vi "Save Data _ Create File.vi"(8 "error in":errorcluster) -> (0 "error out":errorcluster, 1 "FiileNote":string, 2 "FileName":string, 3 "file out":refnum<k34>)   [LabVIEW 2016]
uses:
  Ctrls/GlobeVaribles.vi
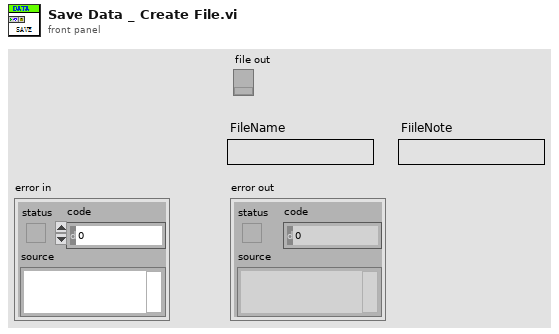
[diagram p1: front panel]
types:
  T1 = enum16{"open", "open or create", "create or replace", "create", "open (read-only)"}
  T2 = typedef "Global para Config.ctl" = cluster{"Timing":cluster{"SampleRate":i32}, "SavePara":cluster{"FlowDiskMode":T3, "SelectMode":T4, "FolderPath":path, "Filename":string, "FileNote":string, "AutoInterval":i32, "Template":path}, "ConfigDS Path*":path, "Tdms Ref*":refnum<k34>}
  T3 = typedef "File Save Mode.ctl" = i32
  T4 = typedef "Select Point Mode.ctl" = i32
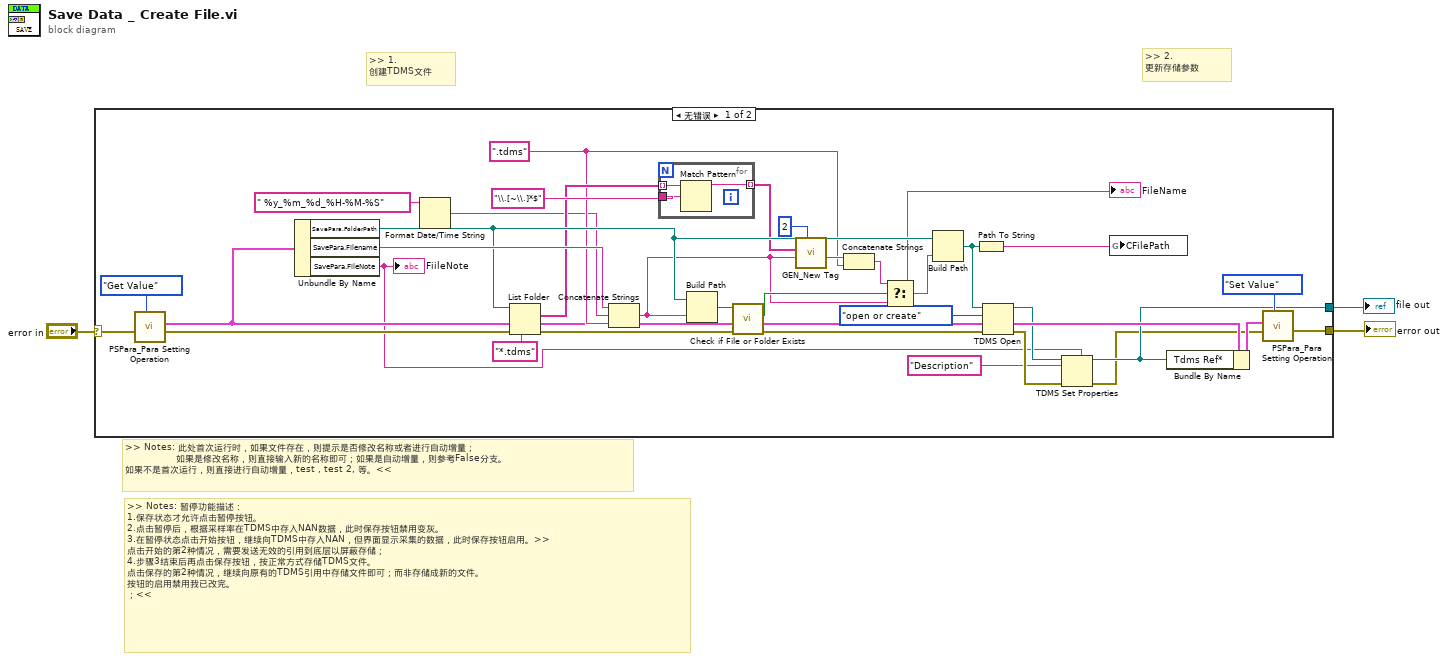
[diagram p0: block diagram]
diagram:
  # ">> 2.\n更新存储参数"
  # ">> 1.\n创建TDMS文件"
  # ">> Notes: 暂停功能描述：\n1.保存状态才允许点击暂停按钮。\n2.点击暂停后，根据采样率在TDMS中存入NAN数据，此时保存按钮禁用变灰。\n3.在暂停状态点击开始按钮，继续向TDMS中存入NAN，但界面显示采集的数据，此时保存按钮启用。>>\n点击开始的第2种情况，需要发送无效的引用到底层以屏蔽存储；\n4.步骤3结束后再点击保存按钮，按正常方式存储TDMS文件。\n点击保存的第2种情况，继续向原有的TDMS引用中存储文件即可；而非存储成新的文件。\n按钮的启用禁用我已改完。\n；<<"
  # ">> Notes: 此处首次运行时，如果文件存在，则提示是否修改名称或者进行自动增量；\n                 如果是修改名称，则直接输入新的名称即可；如果是自动增量，则参考False分支。\n如果不是首次运行，则直接进行自动增量，test , test 2, 等。<<"
  n1 = case shown="无错误" "error in" {
    selector: "error in" -> [w34 w41]
    tunnel: [w37 w41] -> w1
    tunnel: [w8 _] -> w2
    frame No Error {
      w14 = ".tdms" ("字符串")
      n2 = call "PSPara_Para Setting Operation.vi"("Operation"=enum16{"Set Value", "Get Value", "Initialize"}."Get Value", "error in"=w34) -> ("error out"=w33:errorcluster, "_Para"=w10:T2)  [unwired: 8 in]
      n3 = Unbundle By Name(w10) -> ("SavePara.FolderPath"=w35:path, "SavePara.Filename"=w36:string, "SavePara.FileNote"=w5:string)
      "FiileNote" <- w5
      n4 = Format Date/Time String(time format string (%c)=" %y_%m_%d_%H-%M-%S") -> (date/time string=w13:string)  [unwired: 2 in]
      n5 = List Folder(path=w35, pattern="*.tdms", error in=w33) -> (filenames=w24:string[], error out=w16:errorcluster)  [unwired: 1 in, 2 out]
      n6 = Concatenate Strings(w36, w13, w14) -> (w11:string)
      n7 = for {
        tunnel: "\\.[~\\.]*$" ("regular expression") -> [w40]
        tunnel: w24 -> [w39] mode=indexing
        tunnel: [w38] -> w23 mode=indexing
        n8 = Match Pattern(string=w39, regular expression=w40) -> (before substring=w38:string)  [unwired: 4 out]
      }
      n9 = Build Path(base path=w35, name or relative path=w11) -> (appended path=w22:path)
      n10 = call <vilib>:"Check if File or Folder Exists.vi"("error in (no error)"=w16, "path"=w22) -> ("error out"=w15:errorcluster, "file or folder exists?"=w21:bool)  [unwired: 7 in, 1 out]
      n11 = call "GEN_New Tag.vi"("Start Point"=2, "Basic"=w11, "Exist"=w23) -> ("Name"=w29:string)  [unwired: 7 in, 1 out]
      n12 = Concatenate Strings(w29, w14) -> (w20:string)
      n13 = Select(t=w20, s=w21, f=w11) -> (s? t:f=w19:string)
      "FileName" <- w19
      n14 = Build Path(base path=w35, name or relative path=w19) -> (appended path=w18:path)
      n15 = Path To String(path=w18) -> (string=w17:string)
      n16 = TDMS Open(8:w15, 10:T1."open or create" ("operation (0:open)"), 11:w18) -> (0:w7:errorcluster, 3:w9:refnum<k34>)  [unwired: 4 in]
      n17 = TDMS Set Properties(5:w5, 7:"Description", 8:w7, 11:w9) -> (0:w6:errorcluster, 3:w8:refnum<k34>)  [unwired: 2 in, 2 out]
      n18 = global write "GlobeVaribles.vi" "CFilePath"(w17) -> ()
      n19 = Bundle By Name(cluster=w10, "Tdms Ref*"=w8) -> (w31:T2)
      n20 = call "PSPara_Para Setting Operation.vi"("Operation"=enum16{"Set Value", "Get Value", "Initialize"}."Set Value", "error in"=w6, "_Para"=w31) -> ("error out"=w37:errorcluster)  [unwired: 7 in, 1 out]
    }
    frame Error {
    }
  }
  "error out" <- w1
  "file out" <- w2
